vi "p04.vi"() -> ()   [LabVIEW 2015]
panel:
  out "size (in bytes)":i64
  out "data":string
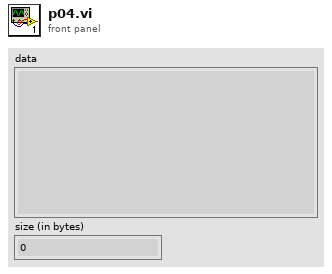
[diagram p1: front panel]
types:
  T1 = enum16{"open", "replace", "create", "open or create", "replace or create", "replace or create with confirmation"}
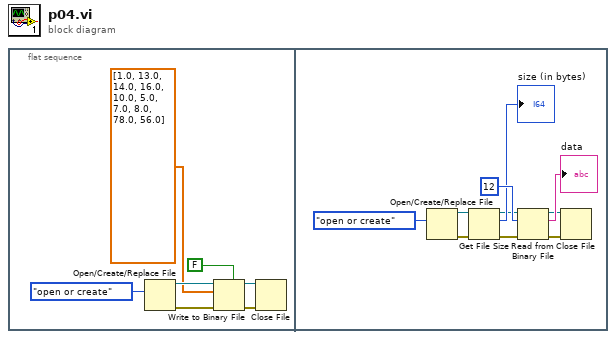
[diagram p0: block diagram]
diagram:
  n1 = flat-sequence {
    frame #0 {
      n2 = Open/Create/Replace File(operation (0:open)=T1."open or create") -> (refnum out=w4:refnum<file>, error out=w6:errorcluster)  [unwired: 5 in, 1 out]
      n3 = Write to Binary File(file (use dialog)=w4, data=dbl[] [1.0, 13.0, 14.0, 16.0, 10.0, 5.0, 7.0, 8.0, 78.0, 56.0] ("Array"), error in=w6, 5:FALSE ("prepend array or string size? (T)")) -> (refnum out=w3:refnum<file>, error out=w5:errorcluster)  [unwired: 2 in, 1 out]
      n4 = Close File(refnum=w3, error in=w5) -> ()  [unwired: 2 out]
    }
    frame #1 {
      n5 = Open/Create/Replace File(operation (0:open)=T1."open or create") -> (refnum out=w12:refnum<file>, error out=w9:errorcluster)  [unwired: 5 in, 1 out]
      n6 = Get File Size(file=w12, error in=w9) -> (refnum out=w13:refnum<file>, size (in bytes)=→"size (in bytes)":i64, 0:w10:errorcluster)
      n7 = Read from Binary File(8:w10, 10:12 ("count (1)"), 11:w13) -> (0:w11:errorcluster, 2:→"data":string, 3:w14:refnum<file>)  [unwired: 3 in, 1 out]
      n8 = Close File(refnum=w14, error in=w11) -> ()  [unwired: 2 out]
    }
  }
